vi "WaitOnProcessSync.vi"(8 "error in (no error)":errorcluster, 9 "timeout in ms (-1)":i32=-1, 11 "JKI SMO in":refnum<class "JKI SMO.lvclass">) -> (0 "error out":errorcluster, 3 "JKI SMO out":refnum<class "JKI SMO.lvclass">)   [LabVIEW 2013, in "JKI SMO.lvclass"]
doc: "This method is used to synchronize processes during launch and shutdown\n\nNote: This method is overridable by descendant\n\n---------------------------------------------------------------\nJKI State Machine Objects™\nhttp://jki.net/state-machine-objects/\nCopyright (C) 2005-2015, JKI <info@jki.net>\nALL RIGHTS RESERVED"
uses:
  JKI SMO.lvclass
  JKI SMO.lvclass/JKI SMO.ctl
panel:
  # "For instructions on how to use the JKI State Machine Objects, examples and video tutorials, visit:\nhttp://jki.net/state-machine-objects/\n\nJKI State Machine Objects™\nhttp://jki.net/state-machine-objects/\nCopyright (C) 2005-2015, JKI <info@jki.net>\nALL RIGHTS RESERVED"
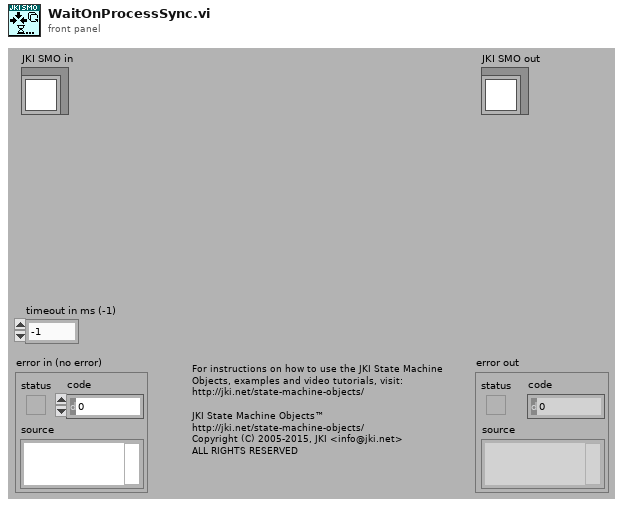
[diagram p1: front panel]
types:
  T1 = typedef "pSubSystem.lvclass/pSubSystem.PrivateData--Cluster.ctl" = cluster{"Processes Clone VI Ref [ ]":refnum<vi>[], "Processes Clone Name [ ]":string[], "Process Sync RendezVous":T2, "Protected Events":T3}
  T2 = typedef "Rendezvous RefNum" = refnum<k1>
  T3 = typedef "pSubSystem.lvclass/pSubSystem.ProtectedEvents--Cluster.ctl" = cluster{"StopProcesses":refnum<user-event>, "AbortProcesses":refnum<user-event>}
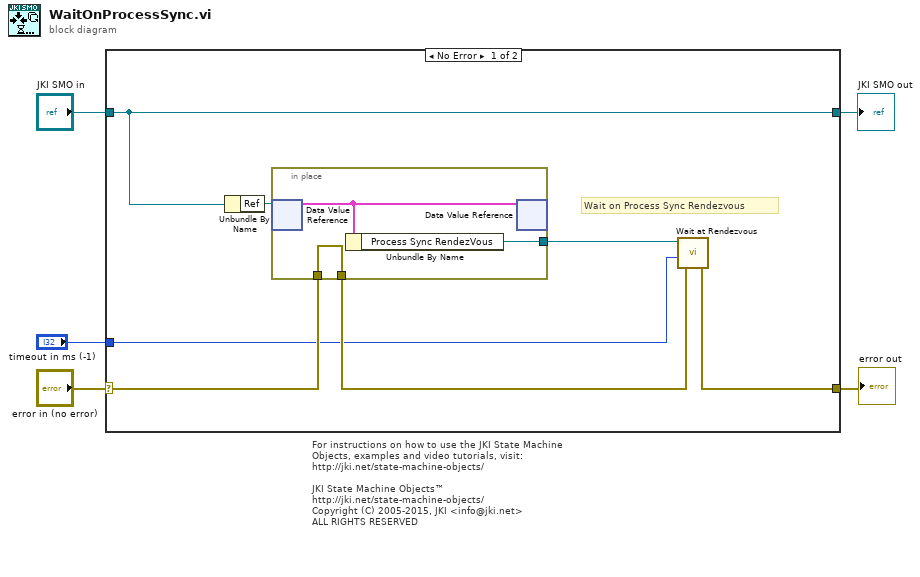
[diagram p0: block diagram]
diagram:
  # "For instructions on how to use the JKI State Machine Objects, examples and video tutorials, visit:\nhttp://jki.net/state-machine-objects/\n\nJKI State Machine Objects™\nhttp://jki.net/state-machine-objects/\nCopyright (C) 2005-2015, JKI <info@jki.net>\nALL RIGHTS RESERVED"
  n1 = case shown="No Error" "error in (no error)" {
    selector: "error in (no error)" -> [w12 w17]
    tunnel: [w10 w17] -> w4
    tunnel: [w6 w16] -> w3
    tunnel: "JKI SMO in" -> [w6 w16]
    tunnel: "timeout in ms (-1)" -> [w9 _]
    frame No Error {
      # "Wait on Process Sync Rendezvous"
      n2 = Unbundle By Name(w6) -> ("Ref"=w8:refnum<data-value>)
      n3 = in-place {
        in-place-border: w12 -> [w15]
        in-place-border: [w15] -> w11
        in-place-border: [w13] -> w7
        n4 = in-place-dvr #1(w8) -> (w14:T1)  [unwired: 1 out]
        n5 = Unbundle By Name(w14) -> ("Process Sync RendezVous"=w13:T2)
        n6 = in-place-dvr #1(w14) -> ()  [unwired: 2 out]
      }
      n7 = call <vilib>:"Wait at Rendezvous.vi"("error in (no error)"=w11, "ms timeout (-1)"=w9, "rendezvous"=w7) -> ("error out"=w10:errorcluster)  [unwired: 4 out]
    }
    frame Error {
    }
  }
  "error out" <- w4
  "JKI SMO out" <- w3
